vi "FindPOSCheckPercentDiff (SubVI).vi"(0 "x":sgl, 1 "y":sgl, 2 "true x":sgl, 3 "true y":sgl, 4 "variation tolerance":sgl) -> (7 "pass x coordinate":bool, 8 "pass y coordinate":bool)   [LabVIEW 2016]
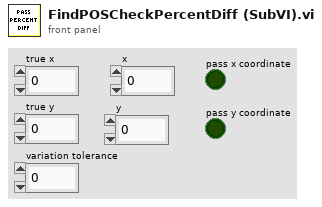
[diagram p1: front panel]
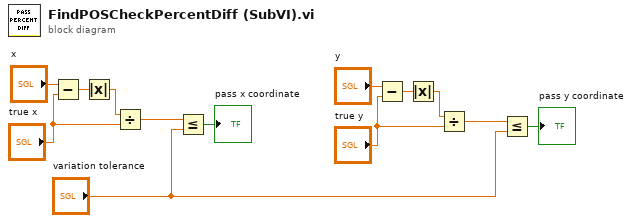
[diagram p0: block diagram]
diagram:
  n1 = Subtract(x="x", y="true x") -> (x-y=w5:sgl)
  n2 = Absolute Value(x=w5) -> (abs(x)=w6:sgl)
  n3 = Divide(x=w6, y="true x") -> (x/y=w7:sgl)
  n4 = Less Or Equal?(x=w7, y="variation tolerance") -> (x <= y?=→"pass x coordinate":bool)
  n5 = Subtract(x="y", y="true y") -> (x-y=w11:sgl)
  n6 = Absolute Value(x=w11) -> (abs(x)=w10:sgl)
  n7 = Divide(x=w10, y="true y") -> (x/y=w9:sgl)
  n8 = Less Or Equal?(x=w9, y="variation tolerance") -> (x <= y?=→"pass y coordinate":bool)
